vi "test_gyro.vi"() -> ()   [LabVIEW 2011]
panel:
  out "error out":errorcluster
  out "Angular Rate":dbl(knob) scale=0.0..10.0
  out "Angle":dbl
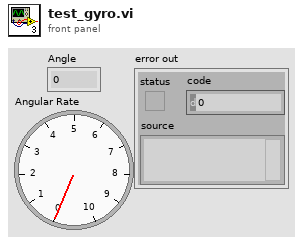
[diagram p1: front panel]
types:
  T1 = typedef "WPI_GyroDevRef.ctl" = cluster{"DevStatus":errorcluster, "Analog Module":T2, "Analog Channel":T3, "Offset":dbl, "Gain (VoltsPerDegree/Second)":dbl}
  T2 = typedef "FPGA_TypedefAnalogModule.ctl" = enum16{"Analog Module 1", "Analog Module 2"}
  T3 = typedef "FPGA_AIChannel.ctl" = enum8{"AI 1", "AI 2", "AI 3", "AI 4", "AI 5", "AI 6", "AI 7", "AI 8", "Invalid"}
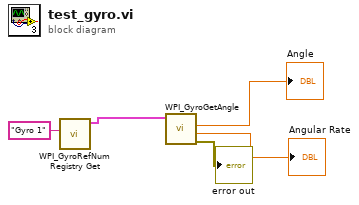
[diagram p0: block diagram]
diagram:
  n1 = call <vilib>:"WPI_GyroRefNum Registry Get.vi"("refnum name"="Gyro 1") -> ("GyroDevRef"=w5:T1)  [unwired: 9 in, 1 out]
  n2 = call <vilib>:"WPI_GyroGetAngle.vi"("GyroDevRef"=w5) -> ("error out"=→"error out":errorcluster, "Angular Rate"=→"Angular Rate":dbl, "Angle"=→"Angle":dbl)  [unwired: 7 in, 1 out]
